vi "Readout.vi"() -> ()   [LabVIEW 2018]
uses:
  <vilib>/Analysis/baseanly.llb/Mean (DBL).vi
  <vilib>/FPGAPlugInAG/myRIO-1900/niLvFpga_Open_myRIO-1900.vi
  <vilib>/rvi/interface/common/dynamic/niFpgaDynamicAddResources.vi
  <vilib>/Utility/error.llb/Error Cluster From Error Code.vi
  <vilib>/rvi/errors/niLvFpgaAdjustHostInterfaceError.vi
  <vilib>/FPGAPlugInAG/Dynamic/niLvFpga_Close_Dynamic.vi
  <vilib>/rvi/interface/nirviOpenFPGA/nirviOpenFPGA.xnode
  FPGA Bitfiles/VoltAmpLoadCellP_FPGATarget_FPGAReadout_bfq+QAGFSf0.lvbitx
  <vilib>/rvi/interface/nirviReadWriteControl/nirviReadWriteControl.xnode
  <vilib>/rvi/interface/nirviCloseFPGA/nirviCloseFPGA.xnode
  NiFpgaLv.dll
  <vilib>/rvi/interface/Simulation/niFpgaSimulationCallBeginRW.vi
  <vilib>/Analysis/NI_AALBase.lvlib
panel:
  out "RawCurrentReading":u16
  in  "Tare 3":bool
  out "LC3 zero point":dbl
  in  "Tare 2":bool
  out "LC2 zero point":dbl
  out "LC3":i32
  out "LC2":i32
  out "50kg Load Cell Chart":dbl(graph)
  out "10kg Load Cell Chart":dbl(graph)
  out "Current Chart 3":dbl(graph)
  out "Current(A)":dbl
  out "LC1 zero point":dbl
  in  "Tare":bool
  out "5kg Load Cell Chart":dbl(graph)
  out "LC1":i32
  out "Voltage Chart":dbl(graph)
  in  "Offset":dbl format="%#_13g"
  in  "Multiplier":dbl=1.0 format="%#_13g"
  out "Voltage (V)":dbl
  in  "Stop":bool
  # "Bem vindo João! Isse é o seu myRIO programa. Você agora pode medir voltage e current."
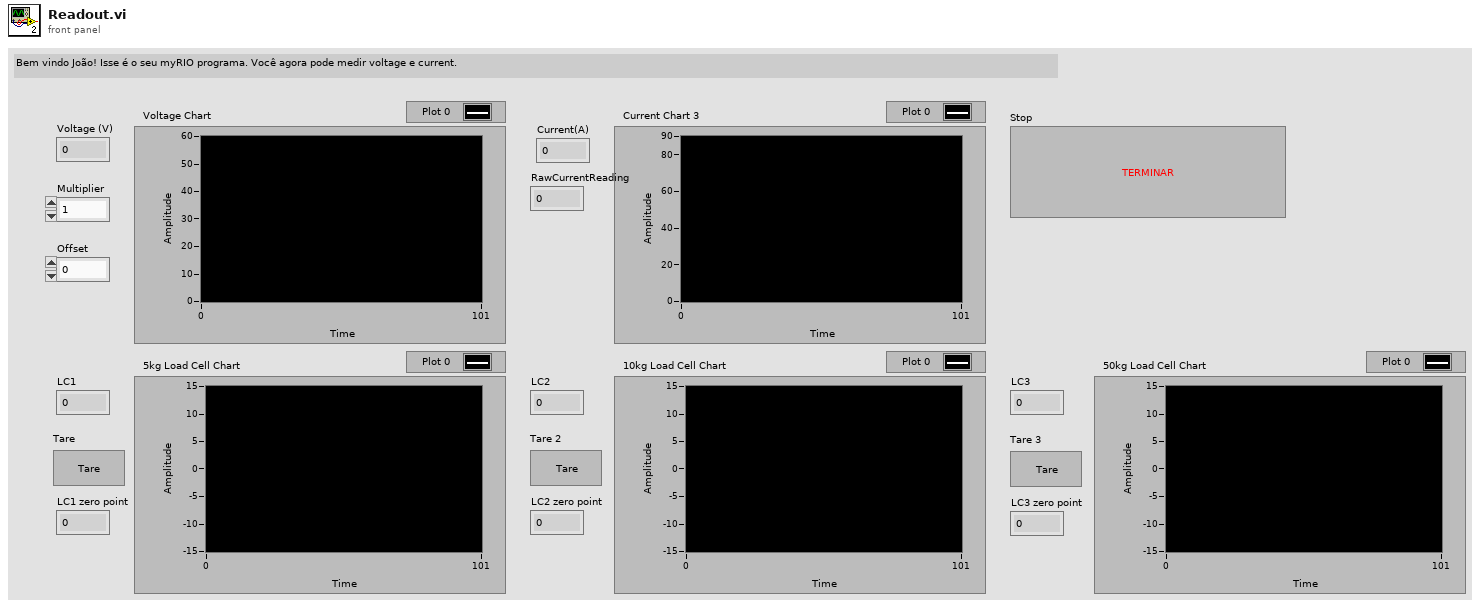
[diagram p1: front panel]
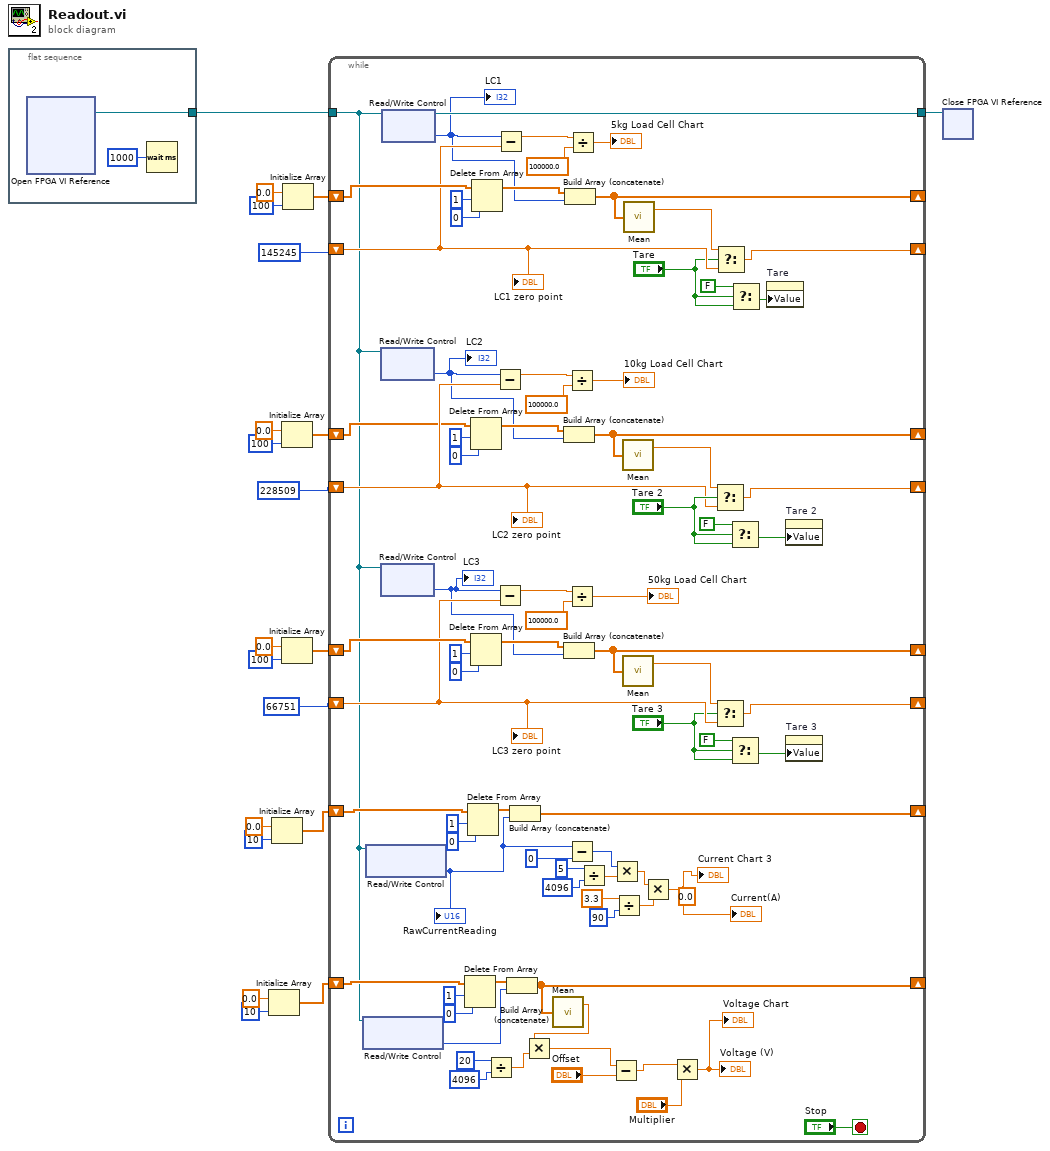
[diagram p0: block diagram]
diagram:
  n1 = flat-sequence {
    tunnel: [w22] -> w20
    frame #0 {
      n2 = xnode "Open FPGA VI Reference"() -> ("FPGA VI Reference Out"=w22:refnum<k20>)  [unwired: 2 in, 1 out]
      n3 = Wait (ms)(milliseconds to wait=u32 1000) -> ()  [unwired: 1 out]
    }
  }
  n4 = Initialize Array(0.0 ("element"), 10 ("dimension size")) -> (w14:dbl[])
  n5 = Initialize Array(0.0 ("element"), 10 ("dimension size")) -> (w9:dbl[])
  n6 = Initialize Array(0.0 ("element"), 100 ("dimension size")) -> (w7:dbl[])
  n7 = Initialize Array(0.0 ("element"), 100 ("dimension size")) -> (w2:dbl[])
  n8 = Initialize Array(0.0 ("element"), 100 ("dimension size")) -> (w16:dbl[])
  n9 = while {
    tunnel: w20 -> [w37]
    tunnel: [w96] -> w19
    shift-right: [w87] -> _
    shift-left: w16 -> [w88]
    shift-right: [w81] -> _
    shift-left: 145245 ("y") -> [w82]
    shift-right: [w71] -> _
    shift-left: w14 -> [w74]
    shift-right: [w69] -> _
    shift-left: w9 -> [w67]
    shift-right: [w57] -> _
    shift-left: w7 -> [w56]
    shift-right: [w62] -> _
    shift-left: 228509 ("y") -> [w61]
    shift-right: [w45] -> _
    shift-left: w2 -> [w46]
    shift-right: [w40] -> _
    shift-left: 66751 ("y") -> [w41]
    stop <- "Stop" stop-if-true
    (unwired) 0.0 ("x*y")
    n10 = xnode "Read/Write Control"("FPGA VI Reference In"=w37) -> ("RawVoltage"=w72:i16)  [unwired: 1 in, 2 out]
    n11 = xnode "Read/Write Control"("FPGA VI Reference In"=w37) -> ("RawCurrent"=w23:u16)  [unwired: 1 in, 2 out]
    "RawCurrentReading" <- w23
    n12 = xnode "Read/Write Control"("FPGA VI Reference In"=w37) -> ("Data 2"=w36:i32)  [unwired: 1 in, 2 out]
    "LC2" <- w36
    n13 = xnode "Read/Write Control"("FPGA VI Reference In"=w37) -> ("Data 3"=w35:i32)  [unwired: 1 in, 2 out]
    "LC3" <- w35
    n14 = xnode "Read/Write Control"("FPGA VI Reference In"=w37) -> ("FPGA VI Reference Out"=w96:refnum<k20>, "Data"=w77:i32)  [unwired: 1 in, 1 out]
    "LC1" <- w77
    n15 = Delete From Array(array=w74, length=1, index=0) -> (array with subset deleted=w73:dbl[])  [unwired: 1 out]
    n16 = Delete From Array(array=w67, length=1, index=0) -> (array with subset deleted=w68:dbl[])  [unwired: 1 out]
    n17 = Delete From Array(array=w56, length=1, index=0) -> (array with subset deleted=w53:dbl[])  [unwired: 1 out]
    n18 = Delete From Array(array=w46, length=1, index=0) -> (array with subset deleted=w49:dbl[])  [unwired: 1 out]
    n19 = Delete From Array(array=w88, length=1, index=0) -> (array with subset deleted=w91:dbl[])  [unwired: 1 out]
    n20 = Divide(x=i16 20, y=i16 4096) -> (x/y=w92:dbl)
    n21 = Subtract(x=w36, y=w61) -> (x-y=w59:dbl)
    n22 = Subtract(x=w35, y=w41) -> (x-y=w43:dbl)
    n23 = Subtract(x=w77, y=w82) -> (x-y=w84:dbl)
    n24 = Build Array (concatenate)(w73, w72) -> (w71:dbl[])
    n25 = Build Array (concatenate)(w68, w23) -> (w69:dbl[])
    n26 = call-poly <vilib>:"Mean.vi"("X"=w71) -> ("mean"=w70:dbl)  [unwired: 1 out]
    n27 = Multiply(x=w70, y=w92) -> (x*y=w95:dbl)
    n28 = Build Array (concatenate)(w53, w36) -> (w57:dbl[])
    n29 = Build Array (concatenate)(w49, w35) -> (w45:dbl[])
    n30 = Build Array (concatenate)(w91, w77) -> (w87:dbl[])
    n31 = Divide(x=w59, y=100000.0) -> (x/y=→"10kg Load Cell Chart":dbl)
    n32 = Divide(x=w43, y=100000.0) -> (x/y=→"50kg Load Cell Chart":dbl)
    n33 = Subtract(x=w23, y=u16 0) -> (x-y=w26:u16)
    n34 = Divide(x=w84, y=100000.0) -> (x/y=→"5kg Load Cell Chart":dbl)
    n35 = Divide(x=i16 5, y=i16 4096) -> (x/y=w30:dbl)
    n36 = Subtract(x=w95, y="Offset") -> (x-y=w99:dbl)
    n37 = Multiply(x=w26, y=w30) -> (x*y=w24:dbl)
    n38 = Divide(x=3.3, y=i16 90) -> (x/y=w27:dbl)
    n39 = call-poly <vilib>:"Mean.vi"("X"=w57) -> ("mean"=w60:dbl)  [unwired: 1 out]
    n40 = call-poly <vilib>:"Mean.vi"("X"=w45) -> ("mean"=w42:dbl)  [unwired: 1 out]
    n41 = call-poly <vilib>:"Mean.vi"("X"=w87) -> ("mean"=w83:dbl)  [unwired: 1 out]
    n42 = Multiply(x=w24, y=w27) -> (x*y=→"Current(A)" →"Current Chart 3":dbl)
    n43 = Multiply(x=w99, y="Multiplier") -> (x*y=→"Voltage (V)" →"Voltage Chart":dbl)
    n44 = Select(t=w60, s="Tare 2", f=w61) -> (s? t:f=w62:dbl)
    n45 = Select(t=w42, s="Tare 3", f=w41) -> (s? t:f=w40:dbl)
    n46 = Select(t=w83, s="Tare", f=w82) -> (s? t:f=w81:dbl)
    n47 = Select(t=FALSE, s="Tare 2", f="Tare 2") -> (s? t:f=w52:bool)
    n48 = Select(t=FALSE, s="Tare 3", f="Tare 3") -> (s? t:f=w50:bool)
    n49 = Select(t=FALSE, s="Tare", f="Tare") -> (s? t:f=w78:bool)
    n50 = property on="Tare" class="Bool"("Value"=w78) -> ()  [unwired: 2 in, 2 out]
    n51 = property on="Tare 2" class="Bool"("Value"=w52) -> ()  [unwired: 2 in, 2 out]
    n52 = property on="Tare 3" class="Bool"("Value"=w50) -> ()  [unwired: 2 in, 2 out]
    "LC1 zero point" <- w82
    "LC2 zero point" <- w61
    "LC3 zero point" <- w41
  }
  n53 = xnode "Close FPGA VI Reference"("FPGA VI Reference In"=w19) -> ()  [unwired: 1 in, 1 out]
